vi "Handle Command.vi"(8 "error in (no error)":errorcluster, 10 "CMD in":refnum<class "Update Chirp CMD.lvclass">, 11 "Object In":refnum<class>) -> (0 "error out":errorcluster, 1 "Command Successful?":bool, 2 "CMD out":refnum<class "Update Chirp CMD.lvclass">, 3 "Object Out":refnum<class>)   [LabVIEW 2018, in "gPAS Library.lvlib" / "Update Chirp CMD.lvclass"]
doc: "This VI will contain the code used to actually execute the request. If the request is successful, this will be indicated by the boolean output <b>Command Successful?</b>. The boolean output can then be used by the <b>Command Reply</b> which sends a reply if the reply queue is valid."
uses:
  Update Chirp CMD.lvclass
  nPAS.lvclass
  C:/Program Files (x86)/National Instruments/LabVIEW 2018/vi.lib/MSR Consulting, LLC/General Reuse/Instrument/Instrument.lvclass
  C:/Program Files (x86)/National Instruments/LabVIEW 2018/vi.lib/MSR Consulting, LLC/General Reuse/PAS/Main/PAS.lvclass
  <vilib>/MSR Consulting, LLC/General Reuse/Instrument/Instrument.lvclass/Instrument.ctl
  nPAS.lvclass/nPAS.ctl
  Update Chirp CMD.lvclass/Update Chirp CMD.ctl
  <vilib>/MSR Consulting, LLC/General Reuse/PAS/Main/PAS.lvclass/PAS.ctl
  <vilib>/MSR Consulting, LLC/General Reuse/PAS/Main/Write Chirp.vi
  <vilib>/MSR Consulting, LLC/General Reuse/Instrument/Read Log Session.vi
  Accessors/Read hFPGA.vi
  <vilib>/MSR Consulting, LLC/General Reuse/Instrument/Read ExtCom.vi
  <vilib>/Utility/error.llb/Error Cluster From Error Code.vi
  <vilib>/rvi/errors/niLvFpgaAdjustHostInterfaceError.vi
  <vilib>/MSR Consulting, LLC/General Reuse/Session APIs/_Session Fwk/Session - Root.lvclass
  <vilib>/rvi/interface/nirviMethod/nirviMethod.xnode
  FPGA Ref.ctl
  FPGA Bitfiles/server.lvbitx
  Session/Raw FPGA/FPGA Session.lvclass
  <vilib>/MSR Consulting, LLC/General Reuse/Session APIs/Session Log/System Log.lvclass
  <vilib>/FPGAPlugInAG/cRIO-9081/niLvFpga_WriteFifo_cRIO-9081.vi
  <vilib>/rvi/errors/niLvFpgaMergeErrorWithErrorCode.vi
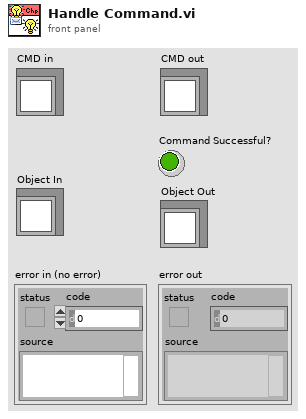
[diagram p1: front panel]
types:
  T1 = typedef "Session - Root.lvclass/Session Handle.ctl" = refnum<data-value>
  T2 = typedef "FPGA Ref.ctl" = refnum<k20>
  T3 = cluster{"tag":string, "section":string, "data":variant}
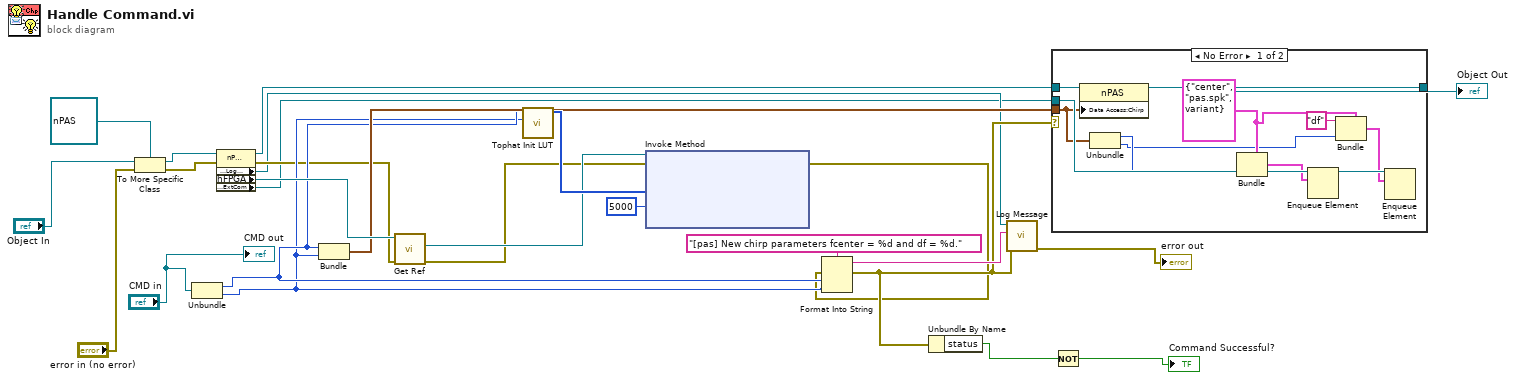
[diagram p0: block diagram]
diagram:
  n1 = To More Specific Class(target class=refnum<class "nPAS.lvclass"> refnum ("nPAS"), reference="Object In", error in="error in (no error)") -> (specific class reference=w24:refnum<class "nPAS.lvclass">, error out=w4:errorcluster)
  n2 = Unbundle("CMD in") -> (w11:i16, w10:i16)
  n3 = property class="nPAS"(reference=w24, error in=w4) -> (reference out=w17:refnum<class "nPAS.lvclass">, error out=w6:errorcluster, "Accessors:Log Session"=w2:T1, "hFPGA"=w23:T1, "Accessors:ExtCom"=w1:refnum<queue>)
  n4 = Bundle("fcenter"=w11, "df"=w10) -> (w15:cluster{"fcenter":i16, "df":i16})  [unwired: 1 in]
  n5 = call "Get Ref.vi"("error in"=w6, "Hanlde Out"=w23) -> ("error out"=w12:errorcluster, "FPGA Ref"=w13:T2)  [unwired: 7 in, 1 out]
  n6 = call <vilib>:"Tophat Init LUT.vi"("Df"=w10, "f0"=w11) -> ("Init Data Out"=w18:i16[])  [unwired: 7 in]
  n7 = xnode "Invoke Method"("FPGA VI Reference In"=w13, "error in"=w12, "Data"=w18, "Timeout (ms)"=5000) -> ("error out"=w7:errorcluster)  [unwired: 2 out]
  n8 = Format Into String(format string="[pas] New chirp parameters fcenter = %d and df = %d.", error in=w7, w11, w10) -> (resulting string=w21:string, error out=w9:errorcluster)  [unwired: 1 in]
  n9 = Unbundle By Name(w9) -> ("status"=w20:bool)
  n10 = call <vilib>:"Log Message.vi"("error in"=w9, "MSG In"=w21, "session in"=w2) -> ("error out"=→"error out":errorcluster)  [unwired: 7 in, 1 out]
  n11 = case shown="No Error" w9 {
    tunnel: w17 -> [w37 w38]
    tunnel: w15 -> [w30 _]
    tunnel: [w36 w38] -> w8
    tunnel: w1 -> [w35 _]
    frame No Error {
      w32 = T3 {"tag"="center", "section"="pas.spk", "data"=variant} ("element")
      n12 = property class="nPAS"(reference=w37, "Data Access:Chirp"=w30) -> (reference out=w36:refnum<class "nPAS.lvclass">)  [unwired: 1 in, 1 out]
      n13 = Unbundle(w30) -> ("fcenter"=w29:i16, "df"=w28:i16)
      n14 = Bundle(cluster=w32, "data"=w29) -> (w34:T3)  [unwired: 2 in]
      n15 = Enqueue Element(queue=w35, element=w34) -> (queue out=w33:refnum<queue>)  [unwired: 2 in, 2 out]
      n16 = Bundle(cluster=w32, "tag"="df", "data"=w28) -> (w27:T3)  [unwired: 1 in]
      n17 = Enqueue Element(queue=w33, element=w27) -> ()  [unwired: 2 in, 3 out]
    }
    frame Error {
    }
  }
  "Object Out" <- w8
  n18 = Not(x=w20) -> (.not. x?=→"Command Successful?":bool)
  "CMD out" <- "CMD in"
